vi "fo_WorklistQuery.vi"(6 "DateRange":T1, 8 "error in (no error)":errorcluster, 11 "ServerInfo":T2={"port"=107, "AEtitle"="MEDIMATIC", "host"="127.0.0.1", "remoteAE"="DVTK_MW_SCP"}) -> (0 "error out":errorcluster, 2 "Result Array":string[][](array[string]), 3 "Tags":string[](array[string]), 5 "Results":refnum<k24>)   [LabVIEW 2013, in "main.lvlib"]
uses:
  main.lvlib
  Controls/Enum Variables.ctl
  C:/Users/Simon/SkyDrive/LabView/2013/DM2020/bin/Dicom.dll
  bin/Dicom.dll
  <userlib>/_MGI/Error Handling/MGI Suppress Error Code/MGI Suppress Error Code (Scalar).vi
panel:
  out "Query Status":string
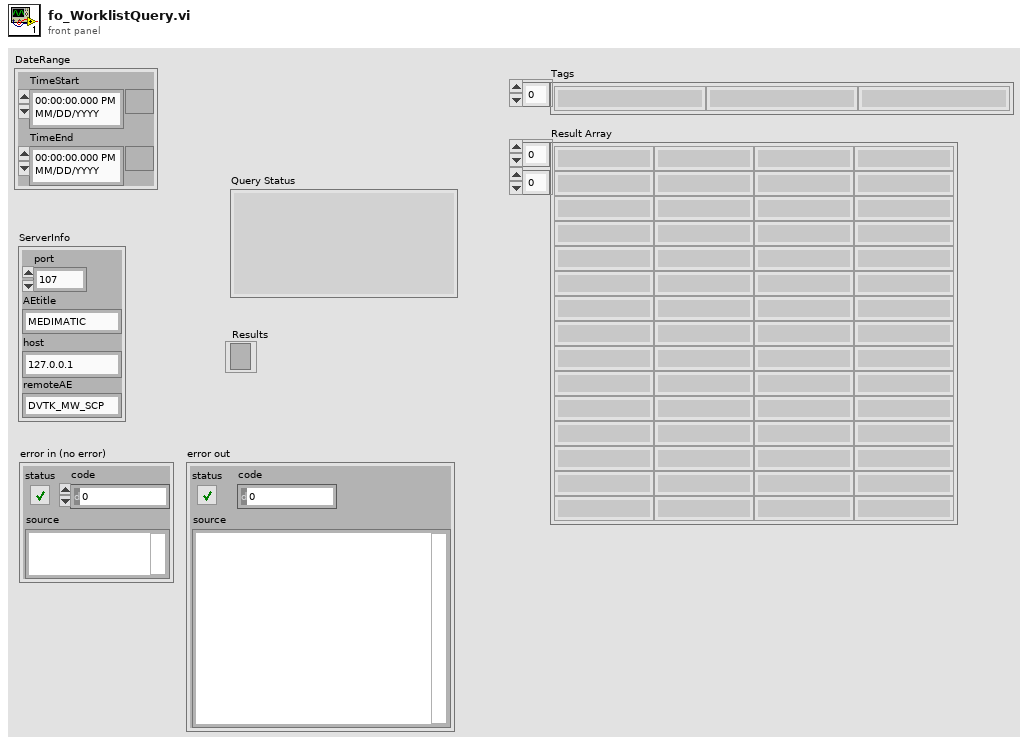
[diagram p1: front panel]
types:
  T1 = cluster{"TimeStart":timestamp, "TimeEnd":timestamp}
  T2 = cluster{"port":i32, "AEtitle":string, "host":string, "remoteAE":string}
  T3 = typedef "main.lvlib/Enum Variables.ctl" = enum16{"SetAcqFilter", "GetAcqFilter", "Set Filter", "Get Filter", "Set Height", "Get Height", "Set Recorded Height", "Get Recorded Height", "Set Blue Pressure", "Get Blue Pressure", "Set Red Pressure", "Get Red Pressure", "Init", "Reset Pressure", "Set Red Cursors", "Get Red Cursors", "Set Blue Cursors", "Get Blue Cursors", "Set Language", "Get Language", "Set Active Graphs", "Get ActiveGraphs", "Set Method", "Get Method", "Set Encryption", "Get Encryption", "Set ExcelVersion", "Get ExcelVersion", "Set DICOM Avail", "Get DICOM Avail", "Set DICOM Encode", "Get DICOM Encode", "Set JournalExport", "Get JournalExport", "Set Sequence", "Get Sequence", "Set DAQ Connected", "Get DAQ Connected", "Set Current Graph", "Get Current Graph", "Set General Settings", "Get Hyphenation", "Set Arm Calc Method", "Get Arm Calc Method", "Set Dicom Tags", "Get Dicom Tags", "Set BT Serial", "Get BT Serial", "Set BT Accepted Serials", "Get BT Accepted Serials", "Get BT License", "Set BT License"}
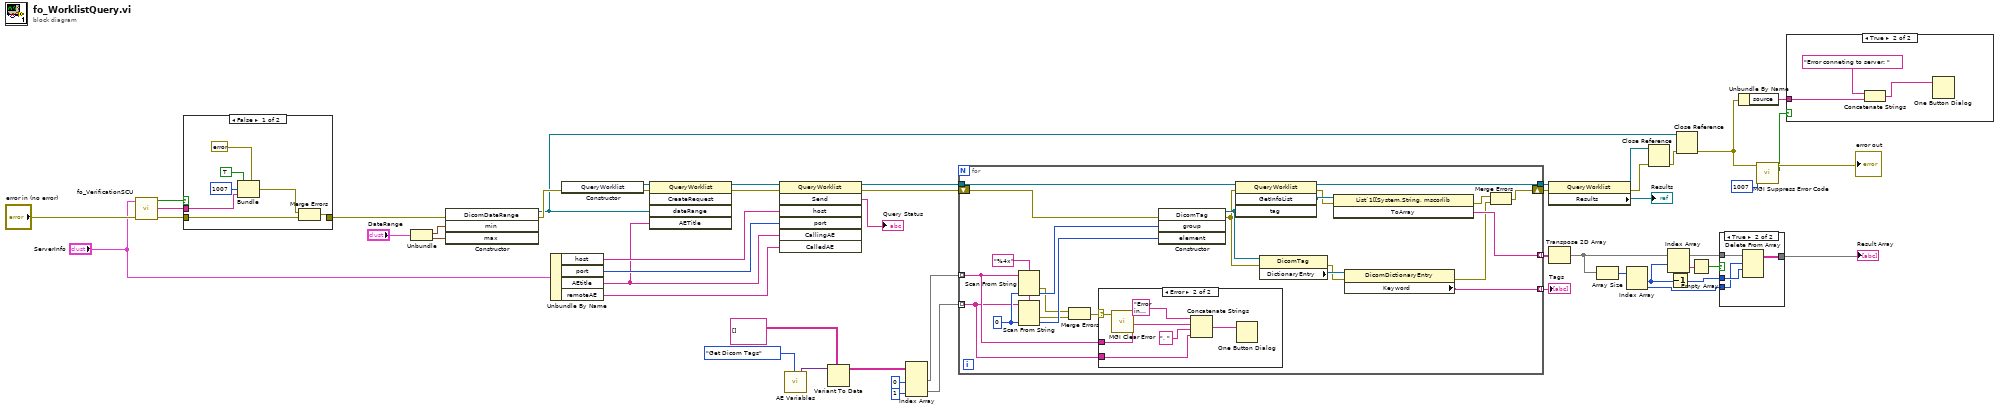
[diagram p0: block diagram]
diagram:
  n1 = call "fo_VerificationSCU.vi"("error in (no error)"="error in (no error)", "ServerInfo"="ServerInfo") -> ("error out"=w16:errorcluster, "status"=w13:string, "Succes?"=w14:bool)  [unwired: 7 in]
  n2 = case shown="False" w14 {
    tunnel: w16 -> [w57 w59]
    tunnel: [w58 w59] -> w15
    tunnel: w13 -> [w53 _]
    frame False {
      n3 = Bundle(cluster=errorcluster {"status"=FALSE, "code"=0, "source"=""} ("error constant"), "status"=TRUE, "code"=1007, "source"=w53) -> (w52:errorcluster)
      n4 = Merge Errors(w52, w57) -> (w58:errorcluster)
    }
    frame True {
    }
  }
  n5 = Unbundle("DateRange") -> ("TimeStart"=w2:timestamp, "TimeEnd"=w1:timestamp)
  n6 = constructor class="DicomDateRange"(error in=w15, "min"=w2, "max"=w1) -> (reference out=w7:refnum<k24>, error out=w39:errorcluster)  [unwired: 2 in, 3 out]
  n7 = Unbundle By Name("ServerInfo") -> ("host"=w48:string, "port"=w47:i32, "AEtitle"=w4:string, "remoteAE"=w46:string)
  n8 = constructor class="QueryWorklist"(error in=w39) -> (reference out=w51:refnum<k24>, error out=w50:errorcluster)  [unwired: 2 in, 1 out]
  n9 = invoke class="QueryWorklist" method="CreateRequest"(reference=w51, error in=w50, "dateRange"=w7, "AETitle"=w4) -> (reference out=w49:refnum<k24>, error out=w44:errorcluster)  [unwired: 1 in, 3 out]
  n10 = invoke class="QueryWorklist" method="Send"(reference=w49, error in=w44, "host"=w48, "port"=w47, "CallingAE"=w4, "CalledAE"=w46) -> (reference out=w45:refnum<k24>, error out=w37:errorcluster, "Send"=→"Query Status":string)  [unwired: 1 in, 4 out]
  n11 = call "AE Variables.vi"("Action"=Enum_Variables."Get Dicom Tags") -> ("Variant"=w33:variant)  [unwired: 11 in, 7 out]
  n12 = Variant To Data(type=string[][] [], Variant=w33) -> (data=w29:string[][])  [unwired: 1 in, 1 out]
  n13 = Index Array(array=w29, index (col) #1=0 ("disabled index (col)"), index (col) #2=1 ("index (col)")) -> (element #1=w31:string[], element #2=w30:string[])  [unwired: 2 in]
  n14 = for {
    tunnel: w45 -> [w82]
    tunnel: [w79] -> w43
    tunnel: w31 -> [w61] mode=indexing
    tunnel: w30 -> [w60] mode=indexing
    tunnel: [w73] -> w36 mode=indexing
    tunnel: [w69] -> w35 mode=indexing
    shift-right: [w67] -> w42
    shift-left: w37 -> [w78]
    w76 = u16 0 ("default value 1")
    w77 = "%4x" ("format string")
    n15 = Scan From String(format string=w77, input string=w61, default 1=w76) -> (error out=w64:errorcluster, output 1=w74:u16)  [unwired: 2 in, 2 out]
    n16 = Scan From String(format string=w77, input string=w60, default 1=w76) -> (error out=w63:errorcluster, output 1=w75:u16)  [unwired: 2 in, 2 out]
    n17 = Merge Errors(w64, w63) -> (w62:errorcluster)
    n18 = case shown="Error" w62 {
      selector: w62 -> [_ w88]
      tunnel: w61 -> [_ w86]
      tunnel: w60 -> [_ w84]
      frame No Error {
      }
      frame Error {
        n19 = call <userlib>:"MGI Clear Error.vi"("Error In"=w88) -> ()  [unwired: 6 in, 1 out]
        n20 = Concatenate Strings("Error in Dicom Tag: " ("message"), w86, ", ", w84) -> (w83:string)
        n21 = One Button Dialog(message=w83) -> ()  [unwired: 1 in, 1 out]
      }
    }
    n22 = constructor class="DicomTag"(error in=w78, "group"=w74, "element"=w75) -> (reference out=w72:refnum<k24>, error out=w68:errorcluster)  [unwired: 2 in, 3 out]
    n23 = invoke class="QueryWorklist" method="GetInfoList"(reference=w82, error in=w68, "tag"=w72) -> (reference out=w79:refnum<k24>, error out=w80:errorcluster, "GetInfoList"=w81:refnum<k24>)  [unwired: 1 in, 1 out]
    n24 = property class="DicomTag"(reference=w72, error in=w68) -> (error out=w70:errorcluster, "DictionaryEntry"=w71:refnum<k24>)  [unwired: 1 out]
    n25 = invoke class="List`1[[System.String, mscorlib" method="ToArray"(reference=w81, error in=w80) -> (error out=w65:errorcluster, "ToArray"=w73:string[])  [unwired: 1 in, 1 out]
    n26 = property class="DicomDictionaryEntry"(reference=w71, error in=w70) -> (error out=w66:errorcluster, "Keyword"=w69:string)  [unwired: 1 out]
    n27 = Merge Errors(w65, w66) -> (w67:errorcluster)
  }
  "Tags" <- w35
  n28 = property class="QueryWorklist"(reference=w43, error in=w42) -> (reference out=w40:refnum<k24>, error out=w41:errorcluster, "Results"=→"Results":refnum<k24>)
  n29 = Transpose 2D Array(2D array=w36) -> (transposed array=w24:string[][])
  n30 = Array Size(array=w24) -> (size(s)=w26:i32[])
  n31 = Index Array(array=w26) -> (element #1=w21:i32, element #2=w19:i32)  [unwired: 2 in]
  n32 = Close Reference(reference=w40, error in (no error)=w41) -> (error out=w8:errorcluster)
  n33 = Index Array(array=w24, index (row)=w21) -> (element=w25:string[])  [unwired: 1 in]
  n34 = Decrement(x=w21) -> (x-1=w20:i32)
  n35 = Close Reference(reference=w7, error in (no error)=w8) -> (error out=w6:errorcluster)
  n36 = Empty Array?(array=w25) -> (empty?=w23:bool)
  n37 = case shown="True" w23 {
    tunnel: w24 -> [w89 w93]
    tunnel: w20 -> [_ w92]
    tunnel: [w89 w91] -> w22
    tunnel: w19 -> [_ w90]
    frame False {
    }
    frame True {
      n38 = Delete From Array(array=w93, length=w90, index (row)=w92) -> (array with subset deleted=w91:string[][])  [unwired: 1 in, 1 out]
    }
  }
  "Result Array" <- w22
  n39 = Unbundle By Name(w6) -> ("source"=w9:string)
  n40 = call-poly <userlib>:"MGI Suppress Error Code.vi"("Error Code"=1007, "Error In"=w6) -> ("Error Supressed?"=w10:bool, "Error Out"=→"error out":errorcluster)  [unwired: 4 in]
  n41 = case shown="True" w10 {
    tunnel: w9 -> [_ w96]
    frame False {
    }
    frame True {
      n42 = Concatenate Strings("Error conneting to server: " ("message"), w96) -> (w94:string)
      n43 = One Button Dialog(message=w94) -> ()  [unwired: 1 in, 1 out]
    }
  }
